vi "Passing Paramters Array Of Integers.vi"(10 "length":i32, 11 "x":i32[](array[numeric])=array[4097 elements]) -> (2 "function return":i32, 3 "x out":i32[](array[numeric]))   [LabVIEW 2018, in "ParsingDataSampleDLL.lvlib"]
doc: "__declspec(dllexport) int PassingParamters_ArrayOfIntegers (int x[], int length);"
uses:
  ParsingDataSampleDLL.lvlib
  ni_reference_vs/Debug/ParsingDataSampleDLL.dll
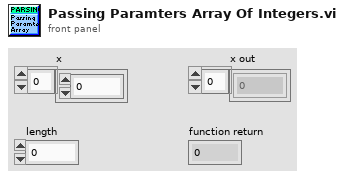
[diagram p1: front panel]
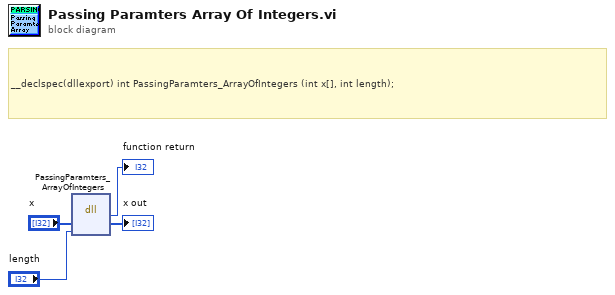
[diagram p0: block diagram]
diagram:
  # "__declspec(dllexport) int PassingParamters_ArrayOfIntegers (int x[], int length);"
  n1 = dll-call lib="C:/Users/celit/Documents/GitHub/Labview_Python_DLL_Call/ni_reference_vs/Debug/ParsingDataSampleDLL.*" fn="PassingParamters_ArrayOfIntegers"("x"="x", "length"="length") -> (→"function return":i32, "x"=→"x out":i32[])  [unwired: 4 in, 2 out]
